vi "ConstructURI.vi"(4 "fragment":string, 6 "query":string, 8 "error in":errorcluster, 9 "path":string, 10 "authority":string, 11 "scheme":string) -> (0 "error out":errorcluster, 3 "URI":string)   [LabVIEW 2013, in "openURI.lvlib"]
uses:
  openURI.lvlib
  URI Components -- cluster.ctl
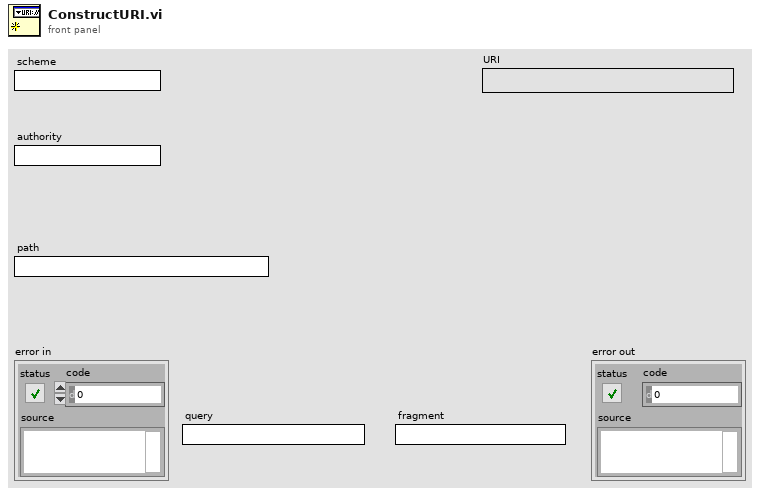
[diagram p1: front panel]
types:
  T1 = typedef "openURI.lvlib/URI Components -- cluster.ctl" = cluster{"scheme":string, "authority":string, "path":string, "query":string, "fragment":string}
  T2 = enum16{"scheme", "authority", "path", "query", "fragment"}
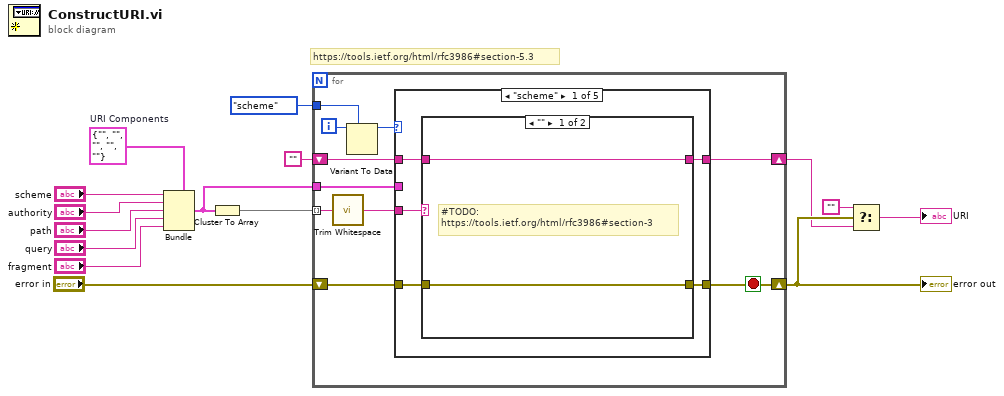
[diagram p0: block diagram]
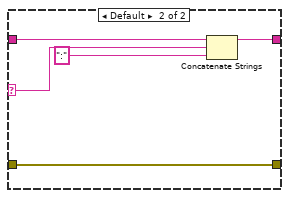
[diagram p2: hidden frame]
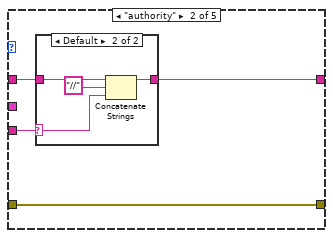
[diagram p3: hidden frame]
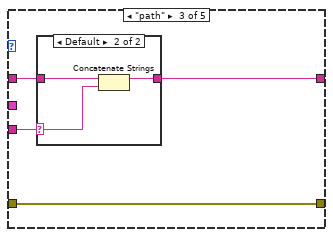
[diagram p5: hidden frame]
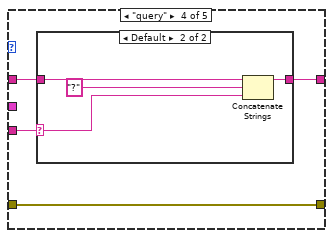
[diagram p7: hidden frame]
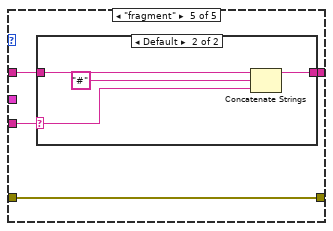
[diagram p9: hidden frame]
diagram:
  w12 = T1 {"scheme"="", "authority"="", "path"="", "query"="", "fragment"=""}  # URI Components
  # "https://tools.ietf.org/html/rfc3986#section-5.3"
  n1 = Bundle(cluster=w12, "scheme"="scheme", "authority"="authority", "path"="path", "query"="query", "fragment"="fragment") -> (w6:T1)
  n2 = Cluster To Array(cluster=w6) -> (array=w7:string[])
  n3 = for {
    tunnel: w7 -> [w23] mode=indexing
    shift-right: [w22] -> w3
    shift-left: "" -> [w24]
    tunnel: T2."scheme" -> [w20]
    tunnel: w6 -> [w18]
    shift-right: [w16] -> w4
    shift-left: "error in" -> [w17]
    i -> [w21]
    stop <- w16 stop-if-true
    n4 = call <vilib>:"Trim Whitespace.vi"("string"=w23) -> ("trimmed string"=w25:string)  [unwired: 1 in]
    n5 = Variant To Data(type=w20, Variant=w21) -> (data=w19:T2)  [unwired: 1 in, 1 out]
    n6 = case shown="\"scheme\"" w19 {
      tunnel: w25 -> [w30 w41 w50 w58 w67]
      tunnel: w24 -> [w29 w40 w49 w57 w66]
      tunnel: [w28 w39 w48 w56 w65] -> w22
      tunnel: w18 -> [_ _ _ _ _]
      tunnel: [w27 w38 w47 w55 w64] -> w16
      tunnel: w17 -> [w26 w38 w47 w55 w64]
      frame "scheme" {
        n7 = case shown="\"\"" w30 {
          selector: w30 -> [_ w36]
          tunnel: w29 -> [w32 w37]
          tunnel: [w32 w34] -> w28
          tunnel: [w31 w33] -> w27
          tunnel: w26 -> [w31 w33]
          frame "" {
            # "#TODO: \nhttps://tools.ietf.org/html/rfc3986#section-3"
          }
          frame Default {
            n8 = Concatenate Strings(w37, w36, ":" ("string")) -> (w34:string)
          }
        }
      }
      frame "authority" {
        n9 = case shown="Default" w41 {
          selector: w41 -> [_ w43]
          tunnel: w40 -> [w42 w46]
          tunnel: [w42 w45] -> w39
          frame "" {
          }
          frame Default {
            n10 = Concatenate Strings(w46, "//" ("string"), w43) -> (w45:string)
          }
        }
      }
      frame "path" {
        n11 = case shown="Default" w50 {
          selector: w50 -> [_ w52]
          tunnel: w49 -> [w51 w54]
          tunnel: [w51 w53] -> w48
          frame "" {
          }
          frame Default {
            n12 = Concatenate Strings(w54, w52) -> (w53:string)
          }
        }
      }
      frame "query" {
        n13 = case shown="Default" w58 {
          selector: w58 -> [_ w60]
          tunnel: w57 -> [w59 w63]
          tunnel: [w59 w62] -> w56
          frame "" {
          }
          frame Default {
            n14 = Concatenate Strings(w63, "?" ("string"), w60) -> (w62:string)
          }
        }
      }
      frame "fragment" {
        n15 = case shown="Default" w67 {
          selector: w67 -> [_ w69]
          tunnel: w66 -> [w68 w72]
          tunnel: [w68 w71] -> w65
          frame "" {
          }
          frame Default {
            n16 = Concatenate Strings(w72, "#" ("string"), w69) -> (w71:string)
          }
        }
      }
    }
  }
  "error out" <- w4
  n17 = Select(t="", s=w4, f=w3) -> (s? t:f=→"URI":string)
